vi "GetParam.vi"(8 "error in (no error)":errorcluster caption="entrée d'erreur (pas d'erreur)", 11 "Precision_Recall_Curve.lvclass":refnum<class "Precision_Recall_Curve.lvclass">) -> (0 "error out":errorcluster caption="sortie d'erreur", 2 "precision_recall_curve":T1={"pos_label"={"dtype_pos_label"="None", "pos_label"="None"}, "sample_weight"=[], "Returns"="precision"}, 3 "Precision_Recall_Curve.lvclass":refnum<class "Precision_Recall_Curve.lvclass">)   [LabVIEW 2020, in "Precision_Recall_Curve.lvclass"]
doc: "Get Parameters"
uses:
  Precision_Recall_Curve.lvclass
  Precision_Recall_Curve.lvclass/Precision_Recall_Curve.ctl
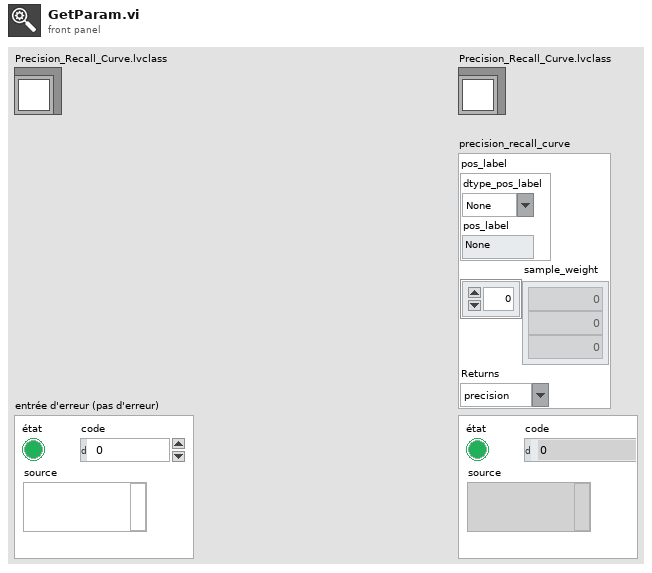
[diagram p1: front panel]
types:
  T1 = cluster{"pos_label":cluster{"dtype_pos_label":string, "pos_label":string}, "sample_weight":dbl[], "Returns":string}
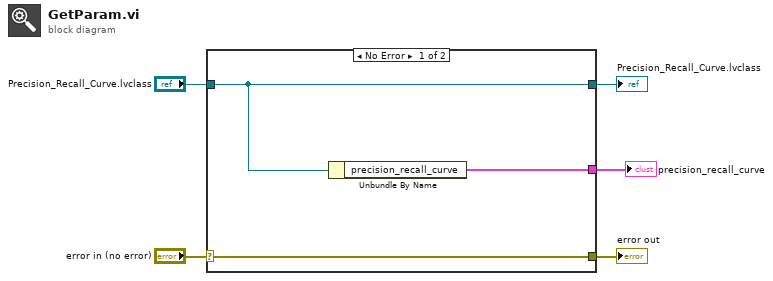
[diagram p0: block diagram]
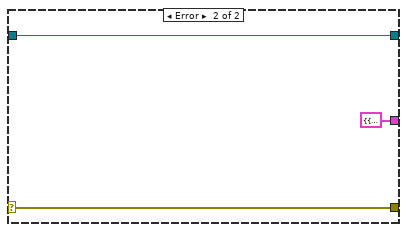
[diagram p2: hidden frame]
diagram:
  n1 = case shown="No Error" "error in (no error)" {
    selector: "error in (no error)" -> [w8 w10]
    tunnel: [w8 w10] -> w4
    tunnel: [w7 w11] -> w2
    tunnel: "Precision_Recall_Curve.lvclass" -> [w7 w11]
    tunnel: [w6 T1 {"pos_label"={"dtype_pos_label"="", "pos_label"=""}, "sample_weight"=[], "Returns"=""} ("precision_recall_curve")] -> w1
    frame No Error {
      n2 = Unbundle By Name(w7) -> ("precision_recall_curve"=w6:T1)
    }
    frame Error {
    }
  }
  "error out" <- w4
  "Precision_Recall_Curve.lvclass" <- w2
  "precision_recall_curve" <- w1
